vi "Teleop.vi"(10 "Match Info":T1={"Autonomous Elapsed Seconds"=0.0, "TeleOp Elapsed Seconds"=0.0, "Disabled Elapsed Seconds"=0.0, "Visited Autonomous"=FALSE, "Visited TeleOp"=FALSE, "Visited Disabled"=FALSE, "Autonomous Settings"={"Autonomous Style"=enum."Independent", "VI Refnum"=refnum}}, 11 "Call Context":T2) -> ()   [LabVIEW 2018]
doc: "This VI is called for each enabled TeleOp packet received from the DS. It is typically used to read from joysticks and other inputs and update I/O or setpoints for timed control loops. It should complete and return within 20 milliseconds or risk missing DS packets."
uses:
  <vilib>/Rock Robotics/WPI/DriverStation/WPI_DriverStationDerivedRobotMode.ctl
  <vilib>/Rock Robotics/WPI/DriverStation/WPI_DriverStationMatch Info.ctl
  <vilib>/Rock Robotics/WPI/Solenoid/WPI_SolenoidValue.ctl
  Framework/Robot Global Data.vi
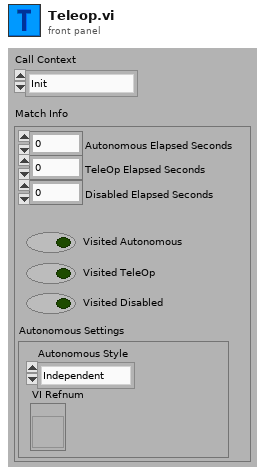
[diagram p1: front panel]
types:
  T1 = typedef "WPI_DriverStationMatch Info.ctl" = cluster{"Autonomous Elapsed Seconds":dbl, "TeleOp Elapsed Seconds":dbl, "Disabled Elapsed Seconds":dbl, "Visited Autonomous":bool, "Visited TeleOp":bool, "Visited Disabled":bool, "Autonomous Settings":cluster{"Autonomous Style":enum16{"Iterative", "Independent"}, "VI Refnum":refnum<vi>}}
  T2 = typedef "WPI_DriverStationDerivedRobotMode.ctl" = enum16{"Init", "Execute", "Stop"}
  T3 = typedef "Command Status Info.ctl" = cluster{"Name":string, "Status":T4, "notifier out":T5}
  T4 = typedef "Completion Status.ctl" = enum16{"Successful", "Aborted", "Incomplete"}
  T5 = typedef "Completion Notifier.ctl" = refnum<notifier>
  T6 = typedef "WPI_SolenoidValue.ctl" = enum16{"Off", "On", "Forward", "Reverse"}
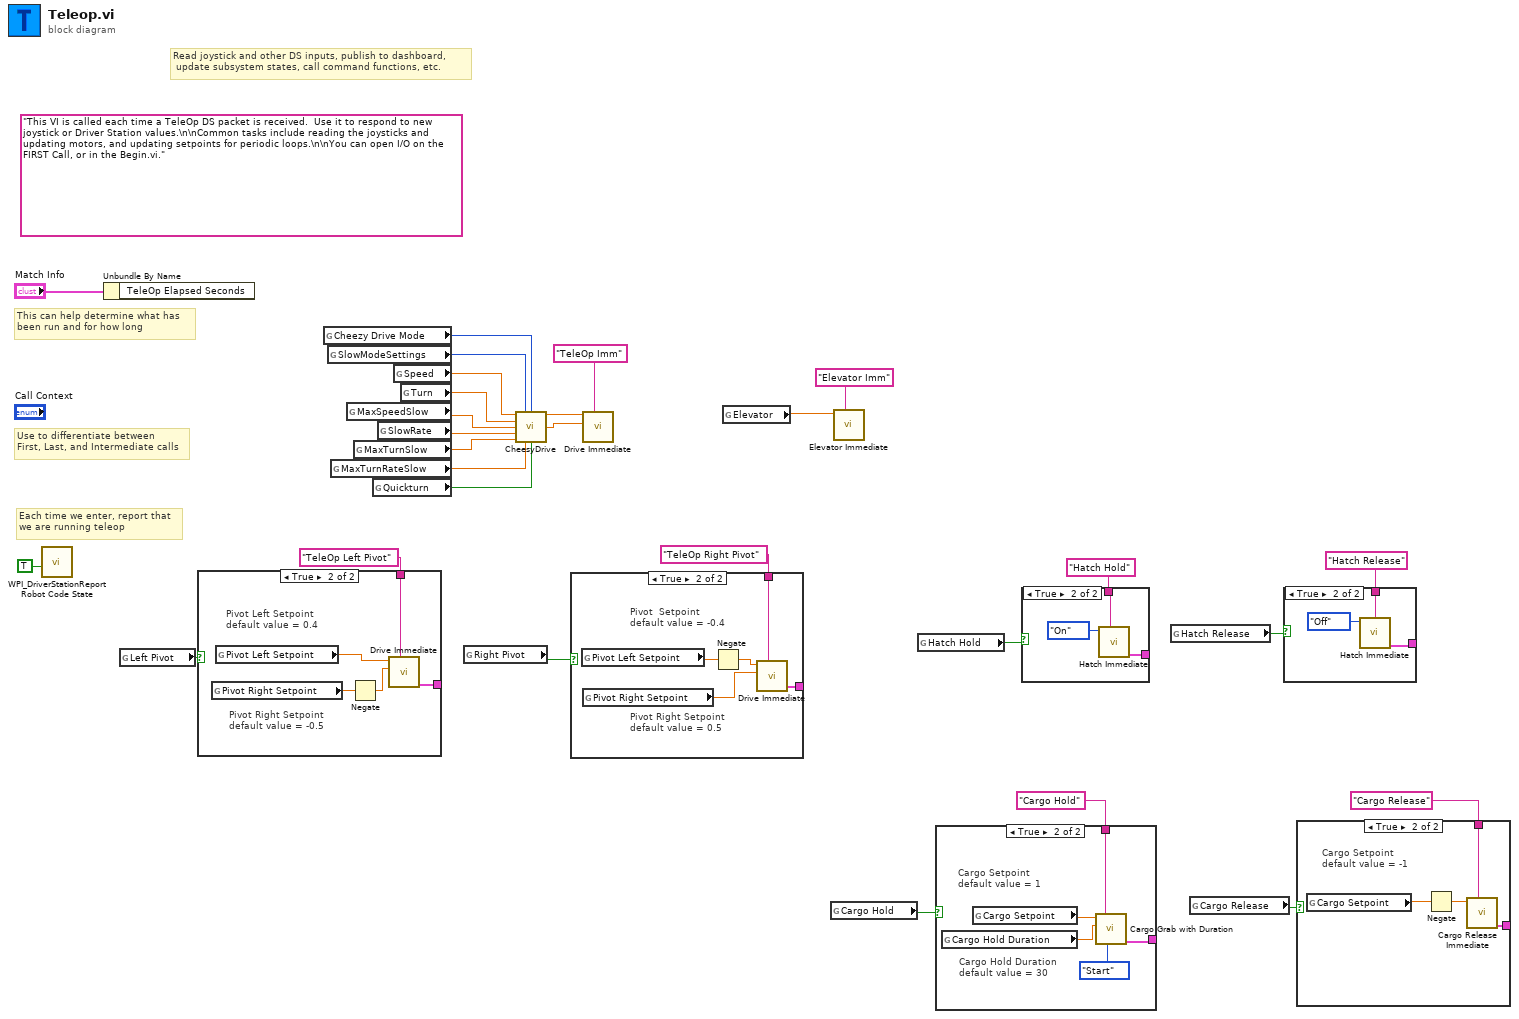
[diagram p0: block diagram]
diagram:
  (unwired) "This VI is called each time a TeleOp DS packet is received.  Use it to respond to new joystick or Driver Station values.\n\nCommon tasks include reading the joysticks and updating motors, and updating setpoints for periodic loops.\n\nYou can open I/O on the FIRST Call, or in the Begin.vi."
  # "Read joystick and other DS inputs, publish to dashboard,\n update subsystem states, call command functions, etc."
  # "Each time we enter, report that\nwe are running teleop"
  # "Use to differentiate between\nFirst, Last, and Intermediate calls"
  # "This can help determine what has\nbeen run and for how long"
  n1 = call <vilib>:"WPI_DriverStationReport Robot Code State.vi"("TeleOp"=TRUE ("Autonomous")) -> ()  [unwired: 10 in, 1 out]
  n2 = Unbundle By Name("Match Info") -> ()  [unwired: 1 out]
  n3 = global read "Robot Global Data.vi" "Left Pivot"() -> (w22:bool)
  n4 = case shown="True" w22 {
    tunnel: [_ w33] -> _
    tunnel: "TeleOp Left Pivot" ("Description") -> [_ w32]
    frame False {
    }
    frame True {
      # "Pivot Right Setpoint\ndefault value = -0.5"
      # "Pivot Left Setpoint\ndefault value = 0.4"
      n5 = global read "Robot Global Data.vi" "Pivot Right Setpoint"() -> (w30:dbl)
      n6 = global read "Robot Global Data.vi" "Pivot Left Setpoint"() -> (w31:dbl)
      n7 = Negate(x=w30) -> (-x=w29:dbl)
      n8 = call "Drive Immediate.vi"("Description"=w32, "Right Setpoint"=w29, "Left Setpoint"=w31) -> ("Command Info Out"=w33:T3)  [unwired: 8 in]
    }
  }
  n9 = global read "Robot Global Data.vi" "Cheezy Drive Mode"() -> (w21:u32)
  n10 = global read "Robot Global Data.vi" "SlowModeSettings"() -> (w11:i32)
  n11 = global read "Robot Global Data.vi" "MaxTurnRateSlow"() -> (w13:dbl)
  n12 = global read "Robot Global Data.vi" "MaxSpeedSlow"() -> (w16:dbl)
  n13 = global read "Robot Global Data.vi" "MaxTurnSlow"() -> (w14:dbl)
  n14 = global read "Robot Global Data.vi" "Quickturn"() -> (w12:bool)
  n15 = global read "Robot Global Data.vi" "SlowRate"() -> (w15:dbl)
  n16 = global read "Robot Global Data.vi" "Speed"() -> (w18:dbl)
  n17 = global read "Robot Global Data.vi" "Turn"() -> (w17:dbl)
  n18 = global read "Robot Global Data.vi" "Right Pivot"() -> (w23:bool)
  n19 = call "CheesyDrive.vi"("Throttle"=w18, "SlowModeSettings"=w11, "SlowMode"=w21, "Wheel"=w17, "MaxSpeedSlow"=w16, "SlowRate"=w15, "MaxTurnSlow"=w14, "MaxTurnRateSlow"=w13, "Quickturn"=w12) -> ("Left PWM"=w20:dbl, "Right PWM"=w19:dbl)  [unwired: 5 in]
  n20 = case shown="True" w23 {
    tunnel: [_ w38] -> _
    tunnel: "TeleOp Right Pivot" ("Description") -> [_ w37]
    frame False {
    }
    frame True {
      # "Pivot Right Setpoint\ndefault value = 0.5"
      # "Pivot  Setpoint\ndefault value = -0.4"
      n21 = global read "Robot Global Data.vi" "Pivot Left Setpoint"() -> (w35:dbl)
      n22 = global read "Robot Global Data.vi" "Pivot Right Setpoint"() -> (w36:dbl)
      n23 = Negate(x=w35) -> (-x=w34:dbl)
      n24 = call "Drive Immediate.vi"("Description"=w37, "Right Setpoint"=w36, "Left Setpoint"=w34) -> ("Command Info Out"=w38:T3)  [unwired: 8 in]
    }
  }
  n25 = call "Drive Immediate.vi"("Description"="TeleOp Imm", "Right Setpoint"=w19, "Left Setpoint"=w20) -> ()  [unwired: 8 in, 1 out]
  n26 = global read "Robot Global Data.vi" "Elevator"() -> (w10:dbl)
  n27 = global read "Robot Global Data.vi" "Cargo Hold"() -> (w6:bool)
  n28 = call "Elevator Immediate.vi"("Description"="Elevator Imm", "Setpoint"=w10) -> ()  [unwired: 9 in, 1 out]
  n29 = global read "Robot Global Data.vi" "Hatch Hold"() -> (w1:bool)
  n30 = case shown="True" w6 {
    tunnel: [_ w43] -> _
    tunnel: "Cargo Hold" ("Description") -> [_ w42]
    frame False {
    }
    frame True {
      # "Cargo Hold Duration\ndefault value = 30"
      # "Cargo Setpoint\ndefault value = 1"
      n31 = global read "Robot Global Data.vi" "Cargo Hold Duration"() -> (w39:dbl)
      n32 = global read "Robot Global Data.vi" "Cargo Setpoint"() -> (w41:dbl)
      n33 = call "Cargo Grab with Duration.vi"("Synchronization"=enum16{"Start", "Wait"}."Start", "Description"=w42, "Duration (s)"=w39, "Setpoint"=w41) -> ("Command Info Out"=w43:T3)  [unwired: 7 in]
    }
  }
  n34 = case shown="True" w1 {
    tunnel: "Hatch Hold" ("Description") -> [_ w46]
    tunnel: [_ w45] -> _
    frame False {
    }
    frame True {
      n35 = call "Hatch Immediate.vi"("Description"=w46, "Relay Value"=WPI_SolenoidValue."On" ("Hatch Action")) -> ("Command Info Out"=w45:T3)  [unwired: 9 in]
    }
  }
  n36 = global read "Robot Global Data.vi" "Hatch Release"() -> (w2:bool)
  n37 = global read "Robot Global Data.vi" "Cargo Release"() -> (w5:bool)
  n38 = case shown="True" w2 {
    tunnel: "Hatch Release" ("Description") -> [_ w49]
    tunnel: [_ w48] -> _
    frame False {
    }
    frame True {
      n39 = call "Hatch Immediate.vi"("Description"=w49, "Relay Value"=WPI_SolenoidValue."Off" ("Hatch Action")) -> ("Command Info Out"=w48:T3)  [unwired: 9 in]
    }
  }
  n40 = case shown="True" w5 {
    tunnel: [_ w53] -> _
    tunnel: "Cargo Release" ("Description") -> [_ w52]
    frame False {
    }
    frame True {
      # "Cargo Setpoint\ndefault value = -1"
      n41 = global read "Robot Global Data.vi" "Cargo Setpoint"() -> (w51:dbl)
      n42 = Negate(x=w51) -> (-x=w50:dbl)
      n43 = call "Cargo Release Immediate.vi"("Description"=w52, "Setpoint"=w50) -> ("Command Info Out"=w53:T3)  [unwired: 9 in]
    }
  }
